vi "ReadLVConfigOptions.vi"(11 "error in":errorcluster) -> (4 "HideIncDec?":bool, 8 "WinPosOffset":T1, 15 "error out":errorcluster)   [LabVIEW 2017, in "Align Elements.lvlib"]
uses:
  Align Elements.lvlib
  <resource>/dialog/lvconfig.llb/LV Config Read Boolean.vi
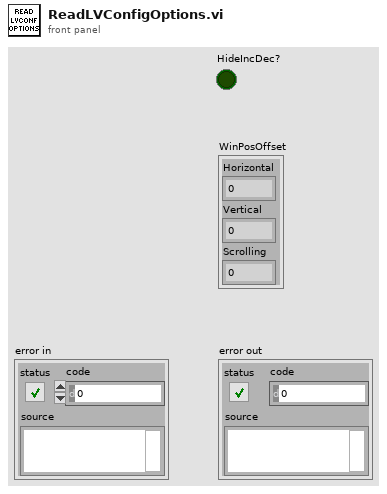
[diagram p1: front panel]
types:
  T1 = cluster{"Horizontal":i32, "Vertical":i32, "Scrolling":i32}
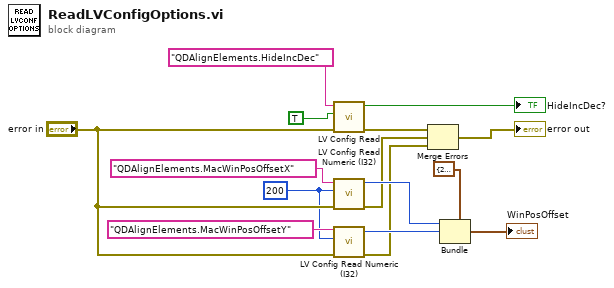
[diagram p0: block diagram]
diagram:
  w8 = 200 ("default value")
  n1 = call-poly <resource>:"LV Config Read.vi"("error in"="error in", "default value"=TRUE, "key"="QDAlignElements.HideIncDec") -> ("error out"=w15:errorcluster, "value"=→"HideIncDec?":bool)  [unwired: 2 in, 1 out]
  n2 = call <resource>:"LV Config Read Numeric (I32).vi"("error in"="error in", "default value"=w8, "key"="QDAlignElements.MacWinPosOffsetX") -> ("error out"=w3:errorcluster, "value"=w6:i32)  [unwired: 2 in, 1 out]
  n3 = call <resource>:"LV Config Read Numeric (I32).vi"("error in"="error in", "default value"=w8, "key"="QDAlignElements.MacWinPosOffsetY") -> ("error out"=w2:errorcluster, "value"=w5:i32)  [unwired: 2 in, 1 out]
  n4 = Merge Errors(w15, w3, w2) -> (→"error out":errorcluster)
  n5 = Bundle(cluster=T1 {"Horizontal"=200, "Vertical"=200, "Scrolling"=0} ("axis info"), "Horizontal"=w6, "Vertical"=w5) -> (→"WinPosOffset":T1)  [unwired: 1 in]
